vi "toJSON.vi"(8 "error in (no error)":errorcluster, 11 "tBSONDouble in":refnum<class "tBSONDouble.lvclass">) -> (0 "error out":errorcluster, 2 "JSON":string, 3 "tBSONDouble out":refnum<class "tBSONDouble.lvclass">)   [LabVIEW 2013, in "BSON.lvlib" / "tBSONDouble.lvclass"]
uses:
  tBSONDouble.lvclass
  tBSONElement/tBSONElement.lvclass
  getValue.vi
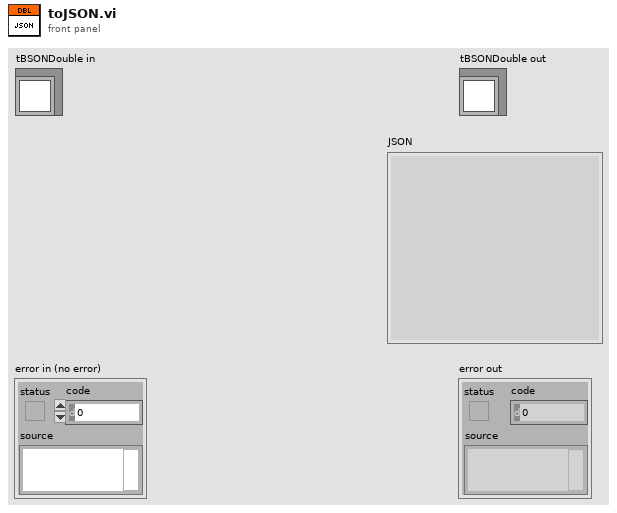
[diagram p1: front panel]
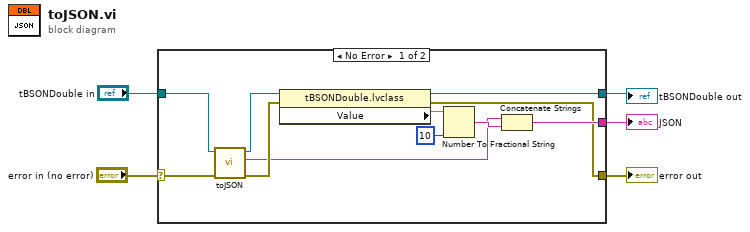
[diagram p0: block diagram]
diagram:
  n1 = case shown="No Error" "error in (no error)" {
    selector: "error in (no error)" -> [w15 w17]
    tunnel: "tBSONDouble in" -> [w16 w18]
    tunnel: [w10 w17] -> w1
    tunnel: [w9 w18] -> w2
    tunnel: [w11 _] -> w3
    frame No Error {
      n2 = call-parent "toJSON.vi"("error in (no error)"=w15, "tBSONElement in"=w16) -> ("error out"=w13:errorcluster, "JSON"=w7:string, "tBSONElement out"=w14:refnum<class "tBSONDouble.lvclass">)  [unwired: 7 in]
      n3 = property class="tBSONDouble.lvclass"(reference=w14, error in=w13) -> (reference out=w9:refnum<class "tBSONDouble.lvclass">, error out=w10:errorcluster, "Value"=w12:dbl)
      n4 = Number To Fractional String(number=w12, precision (6)=i16 10) -> (F-format string=w8:string)  [unwired: 2 in]
      n5 = Concatenate Strings(w7, w8) -> (w11:string)
    }
    frame Error {
    }
  }
  "error out" <- w1
  "tBSONDouble out" <- w2
  "JSON" <- w3
